vi "Public.vi"() -> ()   [LabVIEW 2015, in "Circle Library.lvlib"]
uses:
  Circle Library.lvlib
  Circle cluster.ctl
  colors.ctl
  Shape/Shape.ctl
panel:
  out "output cluster 2":T1
  out "output cluster":T1
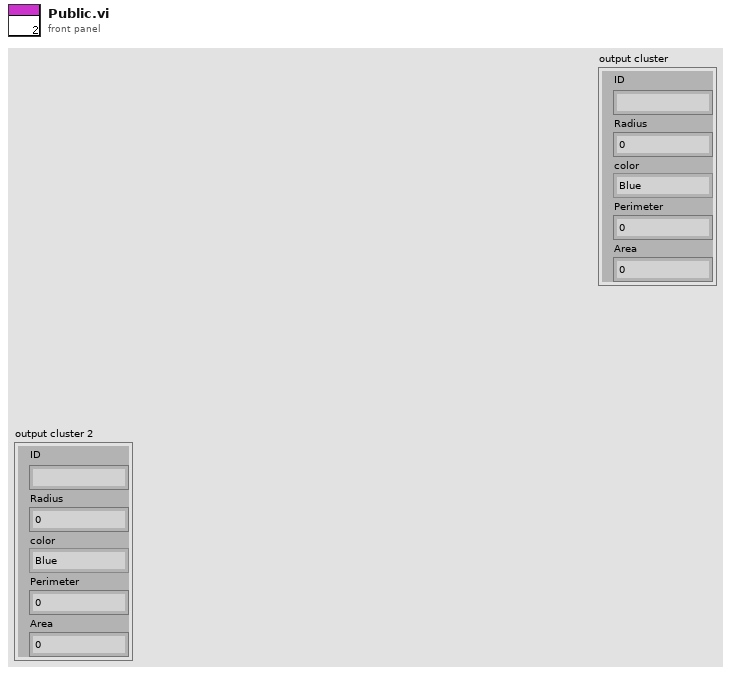
[diagram p1: front panel]
types:
  T1 = typedef "Circle Library.lvlib/Circle cluster.ctl" = cluster{"ID":string, "Radius":dbl, "color":T2, "Perimeter":dbl, "Area":dbl}
  T2 = typedef "colors.ctl" = enum16{"Blue", "Red", "Green", "Yellow"}
  T3 = typedef "Shape.ctl" = enum16{"Square", "Circle"}
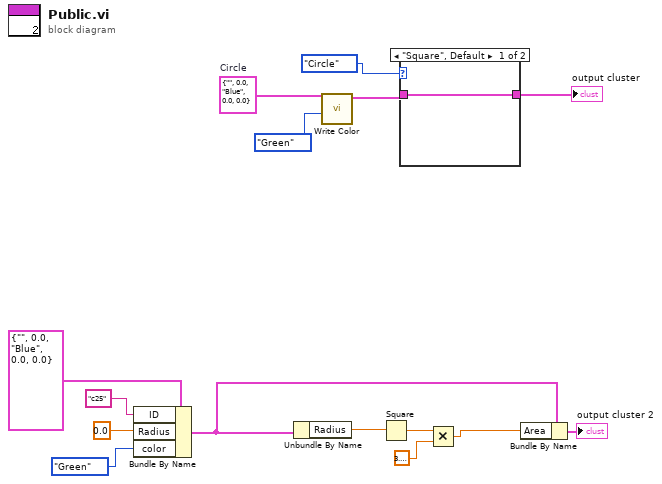
[diagram p0: block diagram]
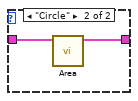
[diagram p2: hidden frame]
diagram:
  w2 = T1 {"ID"="", "Radius"=0.0, "color"=enum."Blue", "Perimeter"=0.0, "Area"=0.0}  # Circle
  n1 = Bundle By Name(cluster=T1 {"ID"="", "Radius"=0.0, "color"=enum."Blue", "Perimeter"=0.0, "Area"=0.0} ("Circle"), "ID"="c25", "Radius"=0.0, "color"=colors."Green") -> (w9:T1)
  n2 = Unbundle By Name(w9) -> ("Radius"=w12:dbl)
  n3 = call "Write Color.vi"("color"=colors."Green", "Circle"=w2) -> ("Circle 2"=w1:T1)  [unwired: 9 in]
  n4 = Square(x=w12) -> (x^2=w11:dbl)
  n5 = case shown="\"Square\", Default" Shape."Circle" {
    tunnel: w1 -> [w16 w18]
    tunnel: [w16 w17] -> w5
    frame "Square", Default {
    }
    frame "Circle" {
      n6 = call "Area.vi"("Circle in"=w18) -> ("Circle Out"=w17:T1)  [unwired: 9 in, 1 out]
    }
  }
  "output cluster" <- w5
  n7 = Multiply(x=w11, y=3.141592653589793) -> (x*y=w8:dbl)
  n8 = Bundle By Name(cluster=w9, "Area"=w8) -> (→"output cluster 2":T1)
